vi "ReadBit.vi"(8 "Error In":errorcluster, 10 "Bit (1-14)":u8=1 min=1 max=14 step=1, 11 "Kiethley 2602 In":refnum<visa-resource-name>) -> (0 "Error Out":errorcluster, 2 "State":bool, 3 "Keithley 2602 Out":refnum<visa-resource-name>)   [LabVIEW 2012, in "Keithley-2602.lvlib"]
uses:
  Keithley-2602.lvlib
panel:
  out "Output":string
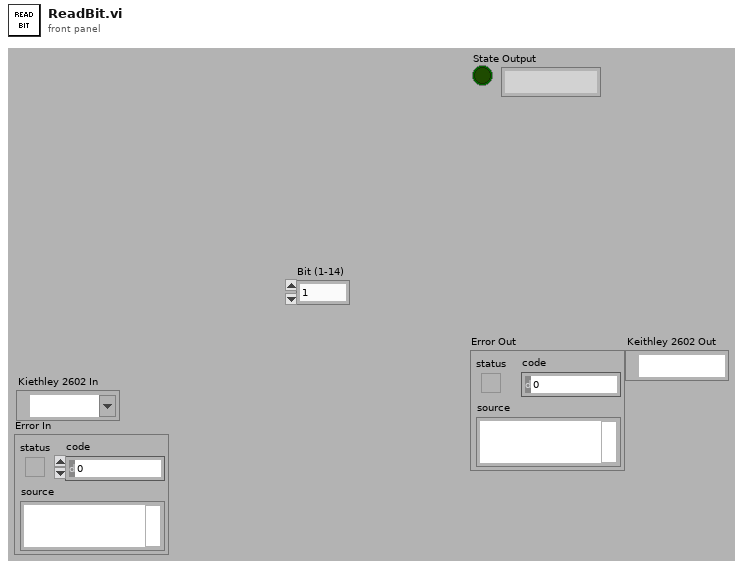
[diagram p1: front panel]
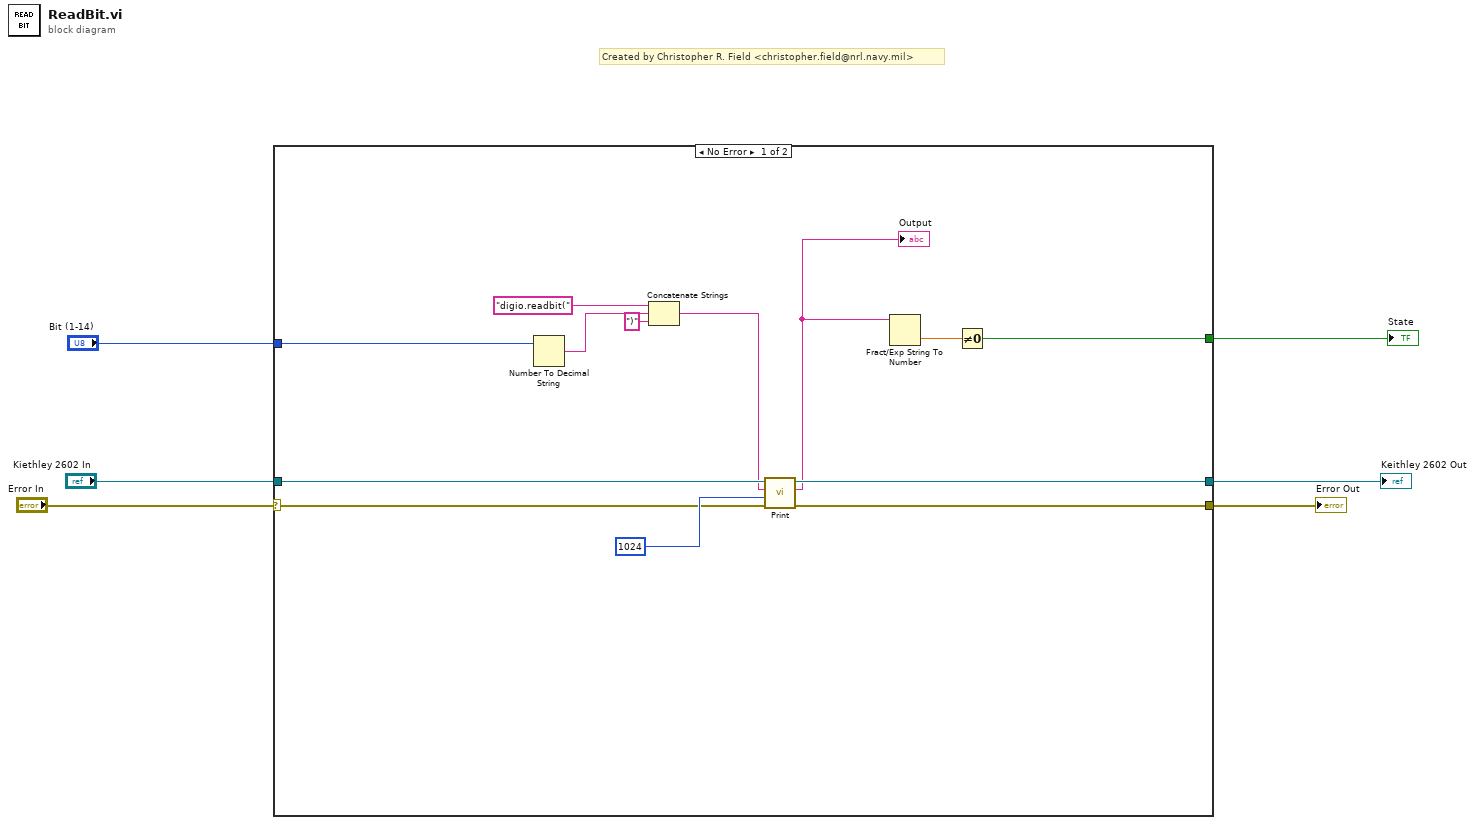
[diagram p0: block diagram]
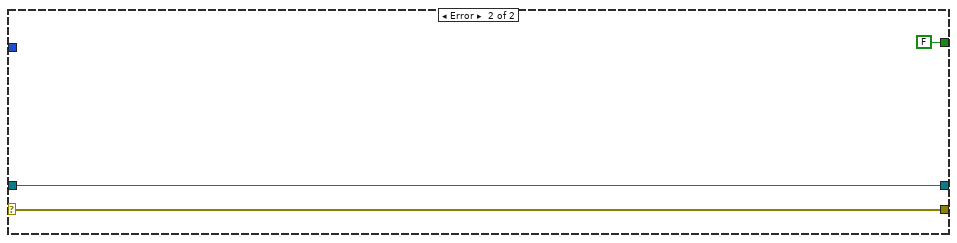
[diagram p2: hidden frame]
diagram:
  # "Created by Christopher R. Field <christopher.field@nrl.navy.mil>"
  n1 = case shown="No Error" "Error In" {
    selector: "Error In" -> [w9 w20]
    tunnel: "Kiethley 2602 In" -> [w18 w21]
    tunnel: [w17 w21] -> w5
    tunnel: [w16 w20] -> w4
    tunnel: "Bit (1-14)" -> [w14 _]
    tunnel: [w11 FALSE] -> w2
    frame No Error {
      n2 = Number To Decimal String(number=w14) -> (decimal integer string=w13:string)  [unwired: 1 in]
      n3 = Concatenate Strings("digio.readbit(", w13, ")" ("string")) -> (w12:string)
      n4 = call "Print.vi"("Error In"=w9, "Byte Count"=u32 1024, "Attribute"=w12, "Kiethley 2602 In"=w18) -> ("Error Out"=w16:errorcluster, "Output"=w8:string, "Keithley 2602 Out"=w17:refnum<visa-resource-name>)  [unwired: 5 in]
      "Output" <- w8
      n5 = Fract/Exp String To Number(string=w8) -> (number=w7:dbl)  [unwired: 3 in, 1 out]
      n6 = Not Equal To 0?(x=w7) -> (x != 0?=w11:bool)
    }
    frame Error {
    }
  }
  "Error Out" <- w4
  "Keithley 2602 Out" <- w5
  "State" <- w2
